vi "set stage range (software).vi"(0 "ASI stage":T1, 5 "x range":dbl, 7 "y range":dbl, 9 "z range":dbl, 11 "error in (no error)":errorcluster) -> (4 "ASI stage out":T1, 15 "error out":errorcluster)   [LabVIEW 2010]
uses:
  stage properties.ctl
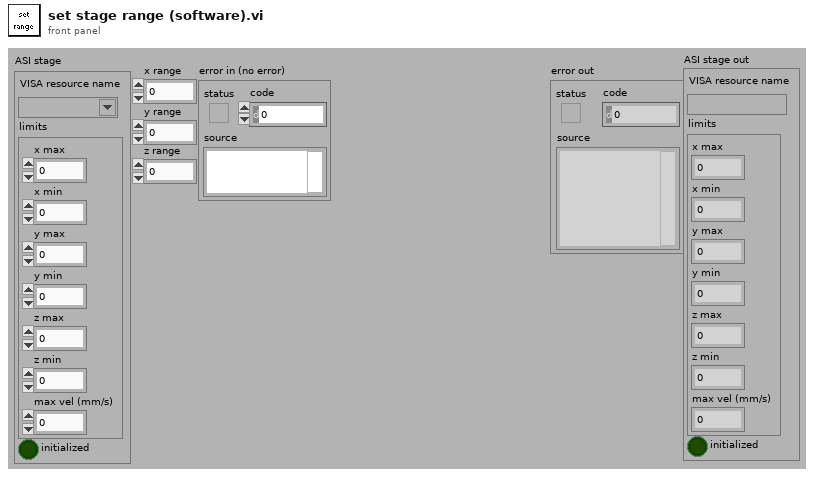
[diagram p1: front panel]
types:
  T1 = typedef "stage properties.ctl" = cluster{"VISA resource name":refnum<visa-resource-name>, "limits":cluster{"x max":dbl, "x min":dbl, "y max":dbl, "y min":dbl, "z max":dbl, "z min":dbl, "max vel (mm/s)":dbl}, "initialized":bool}
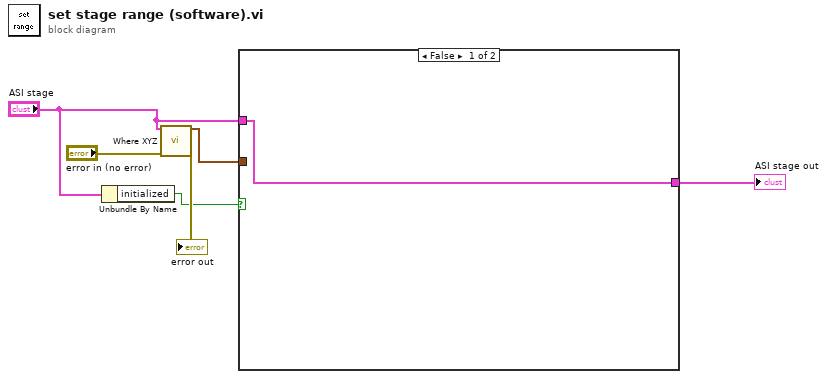
[diagram p0: block diagram]
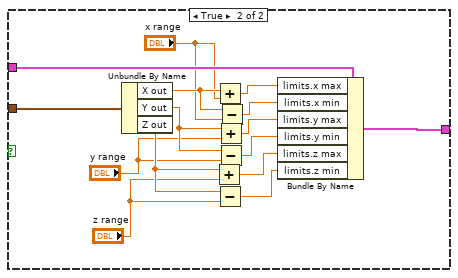
[diagram p2: hidden frame]
diagram:
  n1 = Unbundle By Name("ASI stage") -> ("initialized"=w1:bool)
  n2 = call "Where XYZ.vi"("ASI stage"="ASI stage", "error in (no error)"="error in (no error)") -> ("location"=w6:cluster{"X out":dbl, "Y out":dbl, "Z out":dbl}, "error out"=→"error out":errorcluster)  [unwired: 11 in, 1 out]
  n3 = case shown="False" w1 {
    tunnel: w6 -> [_ w22]
    tunnel: "ASI stage" -> [w7 w21]
    tunnel: [w7 w8] -> w3
    frame False {
    }
    frame True {
      n4 = Unbundle By Name(w22) -> ("X out"=w20:dbl, "Y out"=w19:dbl, "Z out"=w18:dbl)
      n5 = Add(x=w18, y="z range") -> (x+y=w10:dbl)
      n6 = Add(x=w20, y="x range") -> (x+y=w15:dbl)
      n7 = Subtract(x=w18, y="z range") -> (x-y=w9:dbl)
      n8 = Add(x=w19, y="y range") -> (x+y=w13:dbl)
      n9 = Subtract(x=w19, y="y range") -> (x-y=w11:dbl)
      n10 = Subtract(x=w20, y="x range") -> (x-y=w14:dbl)
      n11 = Bundle By Name(cluster=w21, "limits.x max"=w15, "limits.x min"=w14, "limits.y max"=w13, "limits.y min"=w11, "limits.z max"=w10, "limits.z min"=w9) -> (w8:T1)
    }
  }
  "ASI stage out" <- w3
